vi "Send TX Message.vi"(8 "error in (no error)":errorcluster, 11 "RxTx in":refnum<class "CM_RxTx.lvclass">) -> (0 "error out":errorcluster, 3 "RxTx out":refnum<class "CM_RxTx.lvclass">)   [LabVIEW 2018, in "CM_RxTx.lvclass"]
doc: "Send Tx message"
uses:
  CM_RxTx.lvclass
  CM_RxTx.lvclass/CM_RxTx.ctl
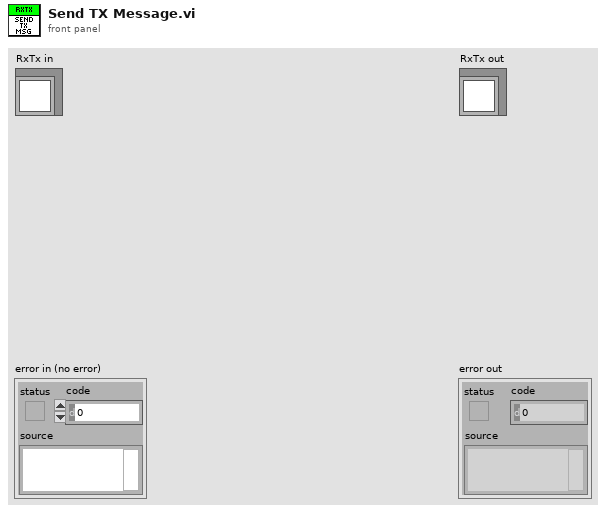
[diagram p1: front panel]
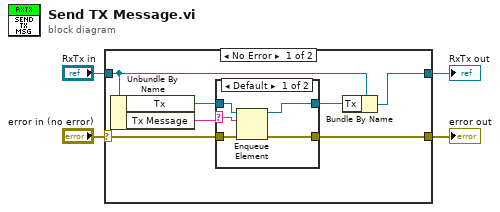
[diagram p0: block diagram]
diagram:
  n1 = case shown="No Error" "error in (no error)" {
    selector: "error in (no error)" -> [w10 w20]
    tunnel: [w9 w20] -> w3
    tunnel: [w6 w19] -> w1
    tunnel: "RxTx in" -> [w7 w19]
    frame No Error {
      n2 = Unbundle By Name(w7) -> ("Tx"=w11:refnum<queue>, "Tx Message"=w8:string)
      n3 = case shown="Default" w8 {
        selector: w8 -> [w13 _]
        tunnel: w11 -> [w16 w17]
        tunnel: w10 -> [w15 w18]
        tunnel: [w14 w18] -> w9
        tunnel: [w12 w17] -> w5
        frame Default {
          n4 = Enqueue Element(queue=w16, element=w13, error in (no error)=w15) -> (queue out=w12:refnum<queue>, error out=w14:errorcluster)  [unwired: 1 in, 1 out]
        }
        frame "" {
        }
      }
      n5 = Bundle By Name(cluster=w7, "Tx"=w5) -> (w6:refnum<class "CM_RxTx.lvclass">)
    }
    frame Error {
    }
  }
  "error out" <- w3
  "RxTx out" <- w1
